vi "Processamento_0310.vi"() -> ()   [LabVIEW 2017]
uses:
  <vilib>/userdefined/High Color/IMAQdx.ctl
  <vilib>/vision/driver/IMAQdx.llb/IMAQdx Acquisition Mode.ctl
  <vilib>/vision/Measure.llb/Straight Edge Options.ctl
  <vilib>/vision/Measure.llb/Straight Edge Process.ctl
  <vilib>/vision/Measure.llb/Edge Options.ctl
  <vilib>/vision/Measure.llb/Edge Polarity.ctl
  <vilib>/vision/driver/IMAQdx.llb/IMAQdx Buffer Number Mode.ctl
  <vilib>/vision/Classification.llb/IMAQ Classifier Read Options.ctl
  <vilib>/vision/NI_Vision_Development_Module.lvlib
  <resource>/objmgr/IMAQImage.rc
  <vilib>/vision/driver/NI_Vision_Acquisition_Software.lvlib
panel:
  out "error out":errorcluster
  in  "Classificador de cor":path
  in  "Stop Button":bool
  in  "Session In":T1
  in  "error in 2":errorcluster
  out "Image Out 2":T2(plugin-control)
  out "Image Out":T2(plugin-control)
types:
  T1 = typedef "IMAQdx.ctl" = refnum<k21>
  T2 = typedef "IMAQ Image.ctl" = refnum<image>
  T3 = typedef "NI_Vision_Acquisition_Software.lvlib/IMAQdx Acquisition Mode.ctl" = enum32{"One Shot", "Continuous"}
  T4 = typedef "Image Type" = u32
  T5 = typedef "NI_Vision_Acquisition_Software.lvlib/IMAQdx Buffer Number Mode.ctl" = enum32{"Next", "Last", "Buffer Number", "Every", "Last New"}
  T6 = typedef "Edge Options.ctl" = cluster{"Edge Polarity":T7, "Kernel Size":u32, "Width":u32, "Minimum Edge Strength":sgl, "Interpolation Type":enum32{"Zero Order", "Bilinear", "Quadratic", "Cubic", "Bilinear Fixed"}, "Data Processing Method":enum32{"Average", "Median"}}
  T7 = typedef "Edge Polarity.ctl" = u32
  T8 = cluster{"Search Direction":u32, "Edge Options":T6, "Show Search Area":bool, "Show Search Lines":bool, "Show Edges Found":bool, "Show Result":bool, "Search Area Color":u32, "Search Lines Color":u32, "Edge Locations Color":u32, "Result Color":u32, "Overlay Group Name":string}
  T9 = cluster{"Objects":u16, "Threshold":i32, "Reject Border":bool, "Fill Holes":bool, "Min Object Size":bool, "Min Size":i32, "Max Object Size":bool, "Max Size":i32, "Show Search Area":bool, "Show Center":bool, "Show Bounding Box":bool}
  T10 = enum32{"AutoM", "Close", "Dilate", "Erode", "Gradient", "Gradient out", "Gradient in", "Hit miss", "Open", "PClose", "POpen", "Thick", "Thin"}
  T11 = cluster{"Desired Font (Application)":enum16{"User-specified Font", "Application Font", "System Font", "Dialog Font"}, "[User-specified Font]":cluster{"Font Name":string, "Size":i16, "Strikeout?":bool, "Italic?":bool, "Underline?":bool, "Outline?":bool, "Shadow?":bool, "Bold?":bool, "Rotation Angle":dbl}, "Horizontal Alignment":i16, "Vertical Alignment":i16}
  T12 = cluster{"Rotation":bool, "Scale":bool, "Occlusion":bool, "Range Settings":cluster{"Match Constraints":u32, "Min":dbl, "Max":dbl}[]}
  T13 = cluster{"Extraction Mode":u32, "Edge Threshold":i32, "Edge Filter Size":u32, "Min Length":i32, "Row Search Step Size":i32, "Col Search Step Size":i32, "Max Endpoint Gap":i32, "Closed":bool, "Subpixel":bool}
  T14 = typedef "Straight Edge Options.ctl" = cluster{"Number of Lines":i32, "Type":T15, "Min. Score":dbl, "Max. Score":dbl, "Orientation":dbl, "Angle Range":dbl, "Angle Tolerance":dbl, "Step Size":u32, "Min. SNR (db)":dbl, "Min. Points (%)":dbl, "Hough Iterations":i32}
  T15 = typedef "Straight Edge Process.ctl" = enum32{"First Edge Rake", "Best Edge Rake", "Hough Edge Rake", "First Edge Projection", "Best Edge Projection"}
  T16 = cluster{"element":dbl, "element":dbl, "x":i32, "y":i32, "element":dbl}
  T17 = typedef "ROI Descriptor" = cluster{"Global Rectangle":i32[], "Contours":cluster{"ID":enum32{"External", "Internal"}, "Type":u32, "Coordinates":i32[]}[]}
  T18 = cluster{"Point1 (Pixels)":cluster{"X":sgl, "Y":sgl}, "Point2 (Pixels)":cluster{"X":sgl, "Y":sgl}, "Point1 (Real-World)":cluster{"X":sgl, "Y":sgl}, "Point2 (Real-World)":cluster{"X":sgl, "Y":sgl}, "Angle (Pixel)":dbl, "Angle (Real-World)":dbl, "Score":dbl, "Straightness":dbl, "Average SNR (db)":dbl, "Calibration Valid":bool}[]
  T19 = cluster{"Point1 (Pixels)":cluster{"X":sgl, "Y":sgl}, "Point2 (Pixels)":cluster{"X":sgl, "Y":sgl}, "Point1 (Real-World)":cluster{"X":sgl, "Y":sgl}, "Point2 (Real-World)":cluster{"X":sgl, "Y":sgl}, "Angle (Pixel)":dbl, "Angle (Real-World)":dbl, "Score":dbl, "Straightness":dbl, "Average SNR (db)":dbl, "Calibration Valid":bool}
  T20 = cluster{"Object Center":cluster{"X":sgl, "Y":sgl}, "Bounding Box":cluster{"X Left":i32, "Y Top":i32, "X Right":i32, "Y Bottom":i32}, "Area":sgl, "Orientation":sgl, "Aspect Ratio":sgl, "Nb Holes":i32}[]
  T21 = cluster{"X Left":i32, "Y Top":i32, "X Right":i32, "Y Bottom":i32}
  T22 = typedef "IMAQ Classifier Read Options.ctl" = i32
  T23 = typedef "IMAQ Classifier Session.ctl" = refnum<k1>
  T24 = cluster{i32, "Object Center":cluster{"X":sgl, "Y":sgl}, "Bounding Box":cluster{"X Left":i32, "Y Top":i32, "X Right":i32, "Y Bottom":i32}, "Number of Matches Returned":i32}
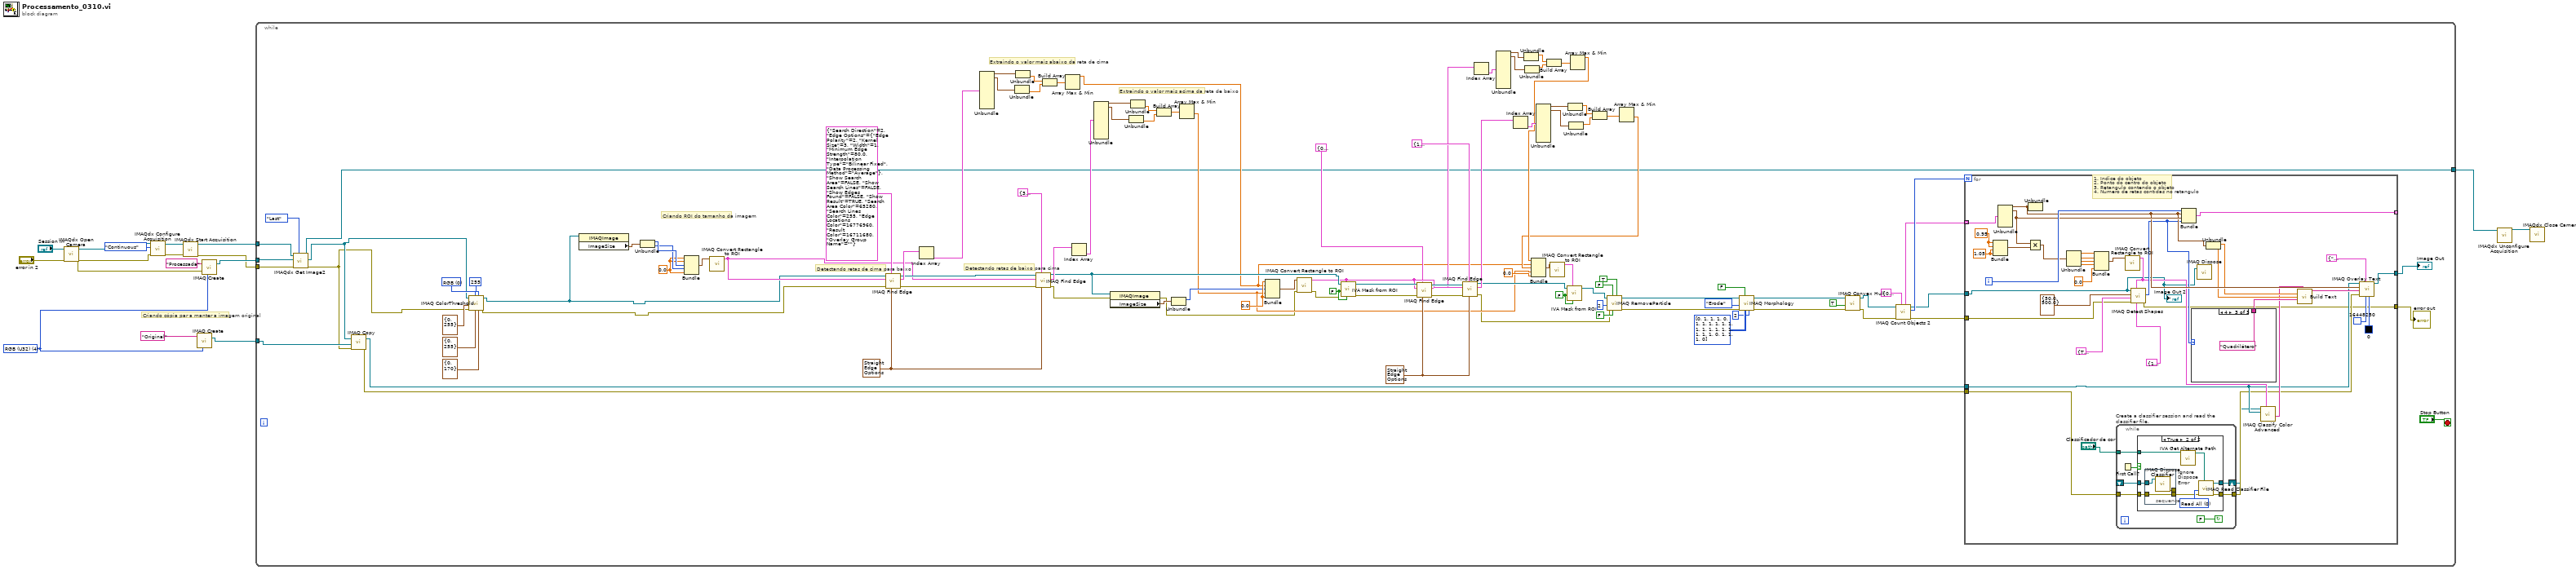
[diagram p0: block diagram]
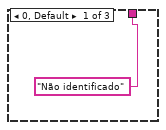
[diagram p3: hidden frame]
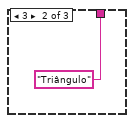
[diagram p4: hidden frame]
diagram:
  w11 = T4 4 items=["Grayscale (U8)", "Grayscale (I16)", "Grayscale (SGL)", "Complex (CSG)", "RGB (U32)", "HSL (U32)", "RGB (U64)", "Grayscale (U16)"] ("Image Type")
  # "Criando cópia par a manter a imagem original"
  n1 = call <vilib>:"IMAQdx Open Camera.vi"("error in"="error in 2", "Session In"="Session In") -> ("error out"=w6:errorcluster, "Session Out"=w9:T1)  [unwired: 1 in, 7 out]
  n2 = call <vilib>:"IMAQdx Configure Acquisition.vi"("error in"=w6, "Continuous?"=IMAQdx_Acquisition_Mode."Continuous", "Session In"=w9) -> ("error out"=w7:errorcluster, "Session Out"=w8:T1)  [unwired: 7 in]
  n3 = call <vilib>:"IMAQdx Start Acquisition.vi"("error in"=w7, "Session In"=w8) -> ("error out"=w5:errorcluster, "Session Out"=w4:T1)  [unwired: 8 in]
  n4 = call "IMAQ Create"("Image Name"="Original", "Image Type"=w11) -> ("New Image"=w15:T2)  [unwired: 3 in, 1 out]
  n5 = call "IMAQ Create"("Image Name"="Processada", "Image Type"=w11, "error in (no error)"=w6) -> ("New Image"=w14:T2)  [unwired: 1 in, 2 out]
  n6 = while {
    tunnel: w15 -> [w24]
    tunnel: w14 -> [w22]
    tunnel: [w18] -> w3
    tunnel: w5 -> [w23]
    tunnel: w4 -> [w21]
    stop <- "Stop Button" stop-if-true
    w39 = u16 0 items=["RGB", "HSL", "HSV", "HSI"] ("Color Mode")
    w72 = FALSE ("Out / In")
    w89 = T14 {"Number of Lines"=1, "Type"=enum."First Edge Rake", "Min. Score"=10.0, "Max. Score"=1000.0, "Orientation"=0.0, "Angle Range"=45.0, "Angle Tolerance"=1.0, "Step Size"=32, "Min. SNR (db)"=0.0, "Min. Points (%)"=25.0, "Hough Iterations"=5} ("Fit Options")
    w94 = FALSE ("Out / In")
    w99 = 0.0
    w96 = 0.0 ("element")
    w90 = T14 {"Number of Lines"=1, "Type"=enum."First Edge Rake", "Min. Score"=10.0, "Max. Score"=1000.0, "Orientation"=0.0, "Angle Range"=45.0, "Angle Tolerance"=1.0, "Step Size"=32, "Min. SNR (db)"=0.0, "Min. Points (%)"=25.0, "Hough Iterations"=5} ("Fit Options")
    # "Extraindo o valor mais acima da reta de baixo"
    # "Extraindo o valor mais abaixo da reta de cima"
    # "Detectando retas de baixo para cima"
    # "Detectando retas de cima para baixo"
    # "Criando ROI do tamanho da imagem"
    n7 = call <vilib>:"IMAQdx Get Image2.vi"("Buffer Number Mode (Next)"=IMAQdx_Buffer_Number_Mode."Last", "error in"=w23, "Image In"=w22, "Session In"=w21) -> ("error out"=w19:errorcluster, "Image Out"=w20:T2, "Session Out"=w18:T1)  [unwired: 4 in, 1 out]
    n8 = call "IMAQ Copy"("error in (no error)"=w19, "Image Dst"=w24, "Image Src"=w20) -> ("error out"=w41:errorcluster, "Image Dst Out"=w48:T2)  [unwired: 3 in]
    n9 = call "IMAQ ColorThreshold"("Blue or Luma or Val or Inten Range"=cluster{"Lower value":i32, "Upper value":i32} {"Lower value"=0, "Upper value"=170}, "Replace Value"=255, "Green or Sat Range"=cluster{"Lower value":i32, "Upper value":i32} {"Lower value"=0, "Upper value"=255}, "Color Mode"=w39, "error in (no error)"=w19, "Red or Hue Range"=cluster{"Lower value":i32, "Upper value":i32} {"Lower value"=0, "Upper value"=255}, "Image Src"=w20) -> ("error out"=w34:errorcluster, "Image Dst Out"=w35:T2)  [unwired: 1 in, 2 out]
    n10 = property class="IMAQImage"(reference=w35) -> ("ImageSize"=w121:cluster{"x":i32, "y":i32})  [unwired: 1 in, 2 out]
    n11 = Unbundle(w121) -> ("x"=w120:i32, "y"=w119:i32)
    n12 = Bundle("element"=w96, "element"=w96, "x"=w120, "y"=w119, "element"=w96) -> (w122:T16)  [unwired: 1 in]
    n13 = call "IMAQ Convert Rectangle to ROI"("Rectangle"=w122) -> ("ROI Descriptor"=w101:T17)  [unwired: 8 in, 1 out]
    n14 = call "IMAQ Find Edge"("Line Fit Options"=w90, "Options"=T8 {"Search Direction"=2, "Edge Options"={"Edge Polarity"=2, "Kernel Size"=3, "Width"=1, "Minimum Edge Strength"=80.0, "Interpolation Type"=enum."Bilinear Fixed", "Data Processing Method"=enum."Average"}, "Show Search Area"=FALSE, "Show Search Lines"=FALSE, "Show Edges Found"=FALSE, "Show Result"=TRUE, "Search Area Color"=65280, "Search Lines Color"=255, "Edge Locations Color"=16776960, "Result Color"=16711680, "Overlay Group Name"=""}, "error in (no error)"=w34, "ROI Descriptor"=w101, "Image"=w35) -> ("error out"=w109:errorcluster, "Straight Edges"=w118:T18, "Image Out"=w110:T2)  [unwired: 1 in, 3 out]
    n15 = Index Array(array=w118) -> (element=w117:T19)  [unwired: 1 in]
    n16 = Unbundle(w117) -> ("Point1 (Pixels)"=w116:cluster{"X":sgl, "Y":sgl}, "Point2 (Pixels)"=w115:cluster{"X":sgl, "Y":sgl})  [unwired: 8 out]
    n17 = Unbundle(w115) -> ("Y"=w113:sgl)  [unwired: 1 out]
    n18 = Unbundle(w116) -> ("Y"=w114:sgl)  [unwired: 1 out]
    n19 = call "IMAQ Find Edge"("Line Fit Options"=w90, "Options"=T8 {"Search Direction"=3, "Edge Options"={"Edge Polarity"=2, "Kernel Size"=3, "Width"=1, "Minimum Edge Strength"=80.0, "Interpolation Type"=enum."Bilinear Fixed", "Data Processing Method"=enum."Average"}, "Show Search Area"=FALSE, "Show Search Lines"=FALSE, "Show Edges Found"=FALSE, "Show Result"=TRUE, "Search Area Color"=65280, "Search Lines Color"=255, "Edge Locations Color"=16776960, "Result Color"=16711680, "Overlay Group Name"=""}, "error in (no error)"=w109, "ROI Descriptor"=w101, "Image"=w110) -> ("error out"=w33:errorcluster, "Straight Edges"=w108:T18, "Image Out"=w95:T2)  [unwired: 1 in, 3 out]
    n20 = Build Array(w114, w113) -> (w112:sgl[])
    n21 = Array Max & Min(array=w112) -> (max value=w65:sgl)  [unwired: 3 out]
    n22 = Index Array(array=w108) -> (element=w102:T19)  [unwired: 1 in]
    n23 = Unbundle(w102) -> ("Point1 (Pixels)"=w103:cluster{"X":sgl, "Y":sgl}, "Point2 (Pixels)"=w104:cluster{"X":sgl, "Y":sgl})  [unwired: 8 out]
    n24 = property class="IMAQImage"(reference=w95, error in=w33) -> (error out=w32:errorcluster, "ImageSize"=w98:cluster{"x":i32, "y":i32})  [unwired: 1 out]
    n25 = Unbundle(w104) -> ("Y"=w106:sgl)  [unwired: 1 out]
    n26 = Unbundle(w103) -> ("Y"=w105:sgl)  [unwired: 1 out]
    n27 = Build Array(w105, w106) -> (w107:sgl[])
    n28 = Unbundle(w98) -> ("x"=w97:i32)  [unwired: 1 out]
    n29 = Array Max & Min(array=w107) -> (min value=w64:sgl)  [unwired: 3 out]
    n30 = Bundle(w99, w65, "x"=w97, w64, w99) -> (w100:cluster{dbl, sgl, "x":i32, sgl, dbl})  [unwired: 1 in]
    n31 = call "IMAQ Convert Rectangle to ROI"("error in (no error)"=w32, "Rectangle"=w100) -> ("error out"=w31:errorcluster, "ROI Descriptor"=w91:T17)  [unwired: 7 in]
    n32 = call <vilib>:"IVA Mask from ROI.vi"("Shrink"=w94, "ROI Descriptor"=w91, "error in (no error)"=w31, "Out / In"=w94, "Image Src"=w95) -> ("error out"=w30:errorcluster, "Image Out"=w93:T2)  [unwired: 5 out]
    n33 = call "IMAQ Find Edge"("Line Fit Options"=w89, "Options"=T8 {"Search Direction"=0, "Edge Options"={"Edge Polarity"=2, "Kernel Size"=3, "Width"=1, "Minimum Edge Strength"=80.0, "Interpolation Type"=enum."Bilinear Fixed", "Data Processing Method"=enum."Average"}, "Show Search Area"=FALSE, "Show Search Lines"=FALSE, "Show Edges Found"=FALSE, "Show Result"=TRUE, "Search Area Color"=65280, "Search Lines Color"=255, "Edge Locations Color"=16776960, "Result Color"=16711680, "Overlay Group Name"=""}, "error in (no error)"=w30, "ROI Descriptor"=w91, "Image"=w93) -> ("error out"=w29:errorcluster, "Straight Edges"=w86:T18, "Image Out"=w92:T2)  [unwired: 1 in, 3 out]
    n34 = call "IMAQ Find Edge"("Line Fit Options"=w89, "Options"=T8 {"Search Direction"=1, "Edge Options"={"Edge Polarity"=2, "Kernel Size"=3, "Width"=1, "Minimum Edge Strength"=80.0, "Interpolation Type"=enum."Bilinear Fixed", "Data Processing Method"=enum."Average"}, "Show Search Area"=FALSE, "Show Search Lines"=FALSE, "Show Edges Found"=FALSE, "Show Result"=TRUE, "Search Area Color"=65280, "Search Lines Color"=255, "Edge Locations Color"=16776960, "Result Color"=16711680, "Overlay Group Name"=""}, "error in (no error)"=w29, "ROI Descriptor"=w91, "Image"=w92) -> ("error out"=w28:errorcluster, "Straight Edges"=w83:T18, "Image Out"=w71:T2)  [unwired: 1 in, 3 out]
    n35 = Index Array(array=w86) -> (element=w85:T19)  [unwired: 1 in]
    n36 = Unbundle(w85) -> ("Point1 (Pixels)"=w82:cluster{"X":sgl, "Y":sgl}, "Point2 (Pixels)"=w81:cluster{"X":sgl, "Y":sgl})  [unwired: 8 out]
    n37 = Index Array(array=w83) -> (element=w84:T19)  [unwired: 1 in]
    n38 = Unbundle(w82) -> ("X"=w78:sgl)  [unwired: 1 out]
    n39 = Unbundle(w81) -> ("X"=w77:sgl)  [unwired: 1 out]
    n40 = Unbundle(w84) -> ("Point1 (Pixels)"=w80:cluster{"X":sgl, "Y":sgl}, "Point2 (Pixels)"=w79:cluster{"X":sgl, "Y":sgl})  [unwired: 8 out]
    n41 = Build Array(w78, w77) -> (w76:sgl[])
    n42 = Unbundle(w80) -> ("X"=w75:sgl)  [unwired: 1 out]
    n43 = Unbundle(w79) -> ("X"=w74:sgl)  [unwired: 1 out]
    n44 = Array Max & Min(array=w76) -> (max value=w67:sgl)  [unwired: 3 out]
    n45 = Build Array(w75, w74) -> (w73:sgl[])
    n46 = Array Max & Min(array=w73) -> (min value=w66:sgl)  [unwired: 3 out]
    n47 = Bundle(w67, w65, w66, w64, 0.0) -> (w69:cluster{sgl, sgl, sgl, sgl, dbl})  [unwired: 1 in]
    n48 = call "IMAQ Convert Rectangle to ROI"("Rectangle"=w69) -> ("ROI Descriptor"=w70:T17)  [unwired: 8 in, 1 out]
    n49 = call <vilib>:"IVA Mask from ROI.vi"("Shrink"=w72, "ROI Descriptor"=w70, "Out / In"=w72, "Image Src"=w71) -> ("Image Out"=w55:T2)  [unwired: 1 in, 6 out]
    n50 = call "IMAQ RemoveParticle"("Connectivity 4/8 (8)"=TRUE, "Low Pass/High Pass (Low)"=FALSE, "Square/Hexa (Square)"=FALSE, "error in (no error)"=w28, "Number of Erosion"=2, "Image Src"=w55) -> ("error out"=w63:errorcluster, "Image Dst Out"=w59:T2)  [unwired: 1 in, 3 out]
    n51 = call "IMAQ Morphology"("Number of iterations (1)"=2, "Structuring Element"=i32[][] [[0, 1, 1, 1, 0], [1, 1, 1, 1, 1], [1, 1, 1, 1, 1], [1, 1, 1, 1, 1], [0, 1, 1, 1, 0]], "Square/Hexa (Square)"=FALSE, "error in (no error)"=w63, "Operation"=T10."Erode", "Image Src"=w59) -> ("error out"=w58:errorcluster, "Image Dst Out"=w57:T2)  [unwired: 1 in, 3 out]
    n52 = call "IMAQ Convex Hull"("error in (no error)"=w58, "Connectivity 4/8 (8)"=TRUE, "Image Src"=w57) -> ("error out"=w27:errorcluster, "Image Dst Out"=w54:T2)  [unwired: 1 in, 6 out]
    n53 = call "IMAQ Count Objects 2"("Settings"=T9 {"Objects"=0, "Threshold"=1, "Reject Border"=FALSE, "Fill Holes"=FALSE, "Min Object Size"=FALSE, "Min Size"=3, "Max Object Size"=FALSE, "Max Size"=100, "Show Search Area"=FALSE, "Show Center"=TRUE, "Show Bounding Box"=TRUE}, "error in (no error)"=w27, "Image"=w54) -> ("error out"=w26:errorcluster, "Number of Objects"=w52:i32, "Image Out"=w50:T2, "Objects"=w51:T20)  [unwired: 4 in, 1 out]
    n54 = for {
      N: w52 -> [_]
      tunnel: w51 -> [w160] mode=indexing
      tunnel: [w158] -> _ mode=indexing
      tunnel: w50 -> [w130]
      tunnel: [w143] -> w49
      tunnel: w48 -> [w131]
      tunnel: w41 -> [w128]
      tunnel: w26 -> [w125]
      tunnel: [w124] -> w25
      i -> [w159]
      w144 = 0.95
      w145 = 1.05
      # "1. Indice do objeto\n2. Ponto do centro do objeto\n3. Retangulo contendo o objeto\n4. Número de retas contidas no retangulo"
      n55 = Bundle(w144, w144, w145, w145) -> (w146:cluster{dbl, dbl, dbl, dbl})  [unwired: 1 in]
      n56 = Unbundle(w160) -> ("Object Center"=w139:cluster{"X":sgl, "Y":sgl}, "Bounding Box"=w148:T21)  [unwired: 4 out]
      n57 = Multiply(x=w148, y=w146) -> (x*y=w147:cluster{dbl, dbl, dbl, dbl})
      n58 = Unbundle(w139) -> ()  [unwired: 2 out]
      n59 = Unbundle(w147) -> (w157:dbl, w156:dbl, w155:dbl, w154:dbl)
      n60 = Bundle(w157, w156, w155, w154, 0.0) -> (w152:cluster{dbl, dbl, dbl, dbl, dbl})  [unwired: 1 in]
      n61 = while "Create a classifier session and read the classifier file." {
        shift-right: [w167] -> w126
        shift-left: _ -> [w166]
        tunnel: w128 -> [w164]
        tunnel: [w163] -> w127
        tunnel: "Classificador de cor" -> [w162]
        stop <- FALSE continue-if-true
        n62 = First Call?() -> (First Call?: T/F=w161:bool)
        n63 = case shown="True" w161 {
          tunnel: [w169 w176] -> w167
          tunnel: w166 -> [w169 w174]
          tunnel: w164 -> [w168 w173]
          tunnel: [w168 w175] -> w163
          tunnel: w162 -> [_ w171]
          frame False {
          }
          frame True {
            w177 = T22 0 items=["Read All", "Add Samples, Do Not Change Options", "Read Options, Do Not Add Samples"] ("Read Options")
            # "Ignore Dispose Error"
            n64 = stacked-sequence {
              tunnel: w174 -> [w180]
              tunnel: w173 -> [w179]
              tunnel: [w179] -> w172
              tunnel: [w178] -> _
              frame #0 {
                n65 = call "IMAQ Dispose Classifier"("Classifier Session"=w180) -> ("error out"=w178:errorcluster)  [unwired: 1 in, 9 out]
              }
            }
            n66 = call <vilib>:"IVA Get Alternate Path.vi"("Path In"=w171) -> ("Path Out"=w170:path)  [unwired: 10 out]
            n67 = call "IMAQ Read Classifier File"("File Path"=w170, "error in (no error)"=w172, "Read Options"=w177) -> ("error out"=w175:errorcluster, "Classifier Session"=w176:T23)  [unwired: 1 in, 6 out]
          }
        }
      }
      n68 = call "IMAQ Convert Rectangle to ROI"("Rectangle"=w152) -> ("ROI Descriptor"=w133:T17)  [unwired: 8 in, 1 out]
      n69 = call-poly "IMAQ Detect Shapes"("Curve Parameters"=T13 {"Extraction Mode"=1, "Edge Threshold"=1, "Edge Filter Size"=1, "Min Length"=50, "Row Search Step Size"=15, "Col Search Step Size"=15, "Max Endpoint Gap"=10, "Closed"=FALSE, "Subpixel"=FALSE}, "ROI Descriptor"=w133, "error in (no error)"=w125, "Match Options"=T12 {"Rotation"=TRUE, "Scale"=FALSE, "Occlusion"=FALSE, "Range Settings"=[{"Match Constraints"=0, "Min"=0.0, "Max"=360.0}]}, "Line Descriptor"=cluster{"Min Length":dbl, "Max Length":dbl} {"Min Length"=50.0, "Max Length"=500.0}, "Image"=w130) -> ("error out"=w124:errorcluster, "Number of Matches Returned"=w136:i32)  [unwired: 3 in, 1 out]
      n70 = Bundle(w159, "Object Center"=w139, "Bounding Box"=w148, "Number of Matches Returned"=w136) -> (w158:T24)  [unwired: 1 in]
      n71 = case shown="4" w136 {
        tunnel: ["Não identificado" "Triângulo" "Quadrilátero"] -> w134
        frame 0, Default {
        }
        frame 3 {
        }
        frame 4 {
        }
      }
      n72 = call "IMAQ Dispose"("Image"=w130) -> ()  [unwired: 5 in, 1 out]
      n73 = Unbundle(w139) -> ("X"=w138:sgl, "Y"=w137:sgl)
      n74 = call "IMAQ Classify Color Advanced"("ROI Descriptor"=w133, "Image"=w131, "Classifier Session"=w126) -> ("Class"=w132:string)  [unwired: 1 in, 7 out]
      n75 = call "Build Text"("cor"=w132, "x"=w138, "y"=w137, "forma"=w134) -> ("Result"=w135:string)  [unwired: 10 in, 1 out]
      n76 = call "IMAQ Overlay Text"("BG Color (Transparent)"=u32 0, "Text Color (black)"=u32 16448250, "Font, Size & Style"=T11 {"Desired Font (Application)"=enum."Application Font", "[User-specified Font]"={"Font Name"="", "Size"=12, "Strikeout?"=FALSE, "Italic?"=FALSE, "Underline?"=FALSE, "Outline?"=FALSE, "Shadow?"=FALSE, "Bold?"=TRUE, "Rotation Angle"=0.0}, "Horizontal Alignment"=1, "Vertical Alignment"=2}, "error in (no error)"=w127, "String"=w135, "Origin"=w139, "Image"=w131) -> ("Image Out"=w143:T2)  [unwired: 3 in, 1 out]
      "Image Out 2" <- w130
    }
    "Image Out" <- w49
    "error out" <- w25
  }
  n77 = call <vilib>:"IMAQdx Unconfigure Acquisition.vi"("Session In"=w3) -> ("Session Out"=w2:T1)  [unwired: 9 in, 1 out]
  n78 = call <vilib>:"IMAQdx Close Camera.vi"("Session In"=w2) -> ()  [unwired: 10 in, 1 out]
